vi "tm_deinitialize.vi"(8 "error in (no error)":errorcluster {"code" format="%.0x"}) -> (0 "error out":errorcluster {"code" format="%.0x"})   [LabVIEW 2012]
uses:
  tmcamcon.dll
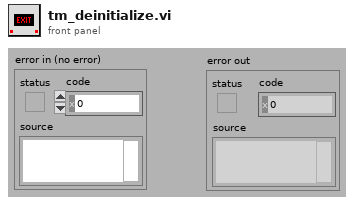
[diagram p1: front panel]
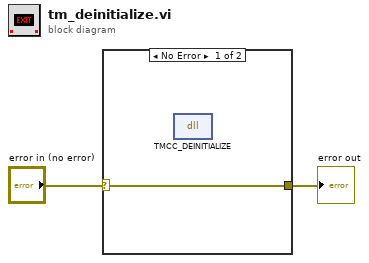
[diagram p0: block diagram]
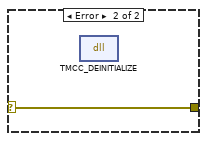
[diagram p2: hidden frame]
diagram:
  n1 = case shown="No Error" "error in (no error)" {
    selector: "error in (no error)" -> [w3 w4]
    tunnel: [w3 w4] -> w2
    frame No Error {
      n2 = dll-call lib="tmcamcon.dll" fn="TMCC_DEINITIALIZE"() -> ()  [unwired: 4 in, 2 out]
    }
    frame Error {
      n3 = dll-call lib="tmcamcon.dll" fn="TMCC_DEINITIALIZE"() -> ()  [unwired: 4 in, 2 out]
    }
  }
  "error out" <- w2
